vi "Teleop.vi"(10 "Match Info":T1={"Autonomous Elapsed Seconds"=0.0, "TeleOp Elapsed Seconds"=0.0, "Disabled Elapsed Seconds"=0.0, "Visited Autonomous"=FALSE, "Visited TeleOp"=FALSE, "Visited Disabled"=FALSE, "Autonomous Settings"={"Autonomous Style"=enum."Independent", "VI Refnum"=refnum}}, 11 "Call Context":T2) -> ()   [LabVIEW 2016]
doc: "This VI is called for each TeleOp packet received from the DS where the robot is not disabled. It is often used to read from the joysticks and update I/O or to update setpoints for timed control loops. It should complete and return within 20 milliseconds or it may miss DS packets."
uses:
  <vilib>/Rock Robotics/WPI/DriverStation/WPI_DriverStationDerivedRobotMode.ctl
  <vilib>/Rock Robotics/WPI/DriverStation/WPI_DriverStationMatch Info.ctl
  <vilib>/Rock Robotics/WPI/Utilities/WPI_GetSetVariantRefNum.vi
  <vilib>/Rock Robotics/Network Tables/NT Write Boolean Array.vi
  <vilib>/Rock Robotics/Network Tables/NT Write Numeric Array.vi
  <vilib>/Rock Robotics/WPI/RobotDrive/WPI_RobotDriveMecanumDrive_Cartesian.vi
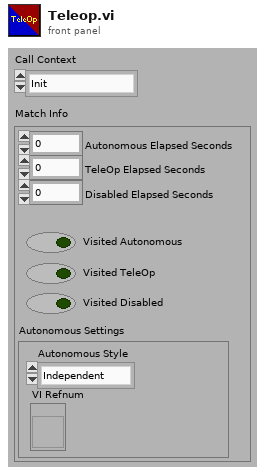
[diagram p1: front panel]
types:
  T1 = typedef "WPI_DriverStationMatch Info.ctl" = cluster{"Autonomous Elapsed Seconds":dbl, "TeleOp Elapsed Seconds":dbl, "Disabled Elapsed Seconds":dbl, "Visited Autonomous":bool, "Visited TeleOp":bool, "Visited Disabled":bool, "Autonomous Settings":cluster{"Autonomous Style":enum16{"Iterative", "Independent"}, "VI Refnum":refnum<vi>}}
  T2 = typedef "WPI_DriverStationDerivedRobotMode.ctl" = enum16{"Init", "Execute", "Stop"}
  T3 = typedef "WPI_JoystickDevRef.ctl" = cluster{"Device":T4}
  T4 = typedef "WPI_JoystickDeviceEnum.ctl" = enum16{"USB 0", "USB 1", "USB 2", "USB 3", "USB 4", "USB 5"}
  T5 = typedef "WPI_RobotDriveDevRef.ctl" = cluster{"DevStatus":errorcluster, "Motors[]":T6[], "Square Inputs":bool, "Max Output":dbl}
  T6 = typedef "WPI_MotorControlDeviceRef.ctl" = cluster{"DeviceStatus":errorcluster, "Type":T7, "PWM":cluster{"PWM Channel":T8, "DeadBand":T9}, "CAN":cluster{"Device Number":u8, "SetOutput VI Ref":variant, "GetOutput VI Ref":variant, "Enable VI Ref":variant, "Disable VI Ref":variant, "Data":variant}, "Invert":bool}
  T7 = typedef "WPI_MotorControlType.ctl" = enum16{"PWM", "CAN"}
  T8 = typedef "FPGA_DIOPWMChannel.ctl" = enum8{"PWM 0", "PWM 1", "PWM 2", "PWM 3", "PWM 4", "PWM 5", "PWM 6", "PWM 7", "PWM 8", "PWM 9", "PWM MXP 0", "PWM MXP 1", "PWM MXP 2", "PWM MXP 3", "PWM MXP 4", "PWM MXP 5", "PWM MXP 6", "PWM MXP 7", "PWM MXP 8", "PWM MXP 9", "Invalid"}
  T9 = typedef "WPI_PWMDeadband.ctl" = cluster{"Name":string, "maxPositivePwm":i32, "minPositivePwm":i32, "centerPwm":i32, "maxNegativePwm":i32, "minNegativePwm":i32, "angularRange":u16}
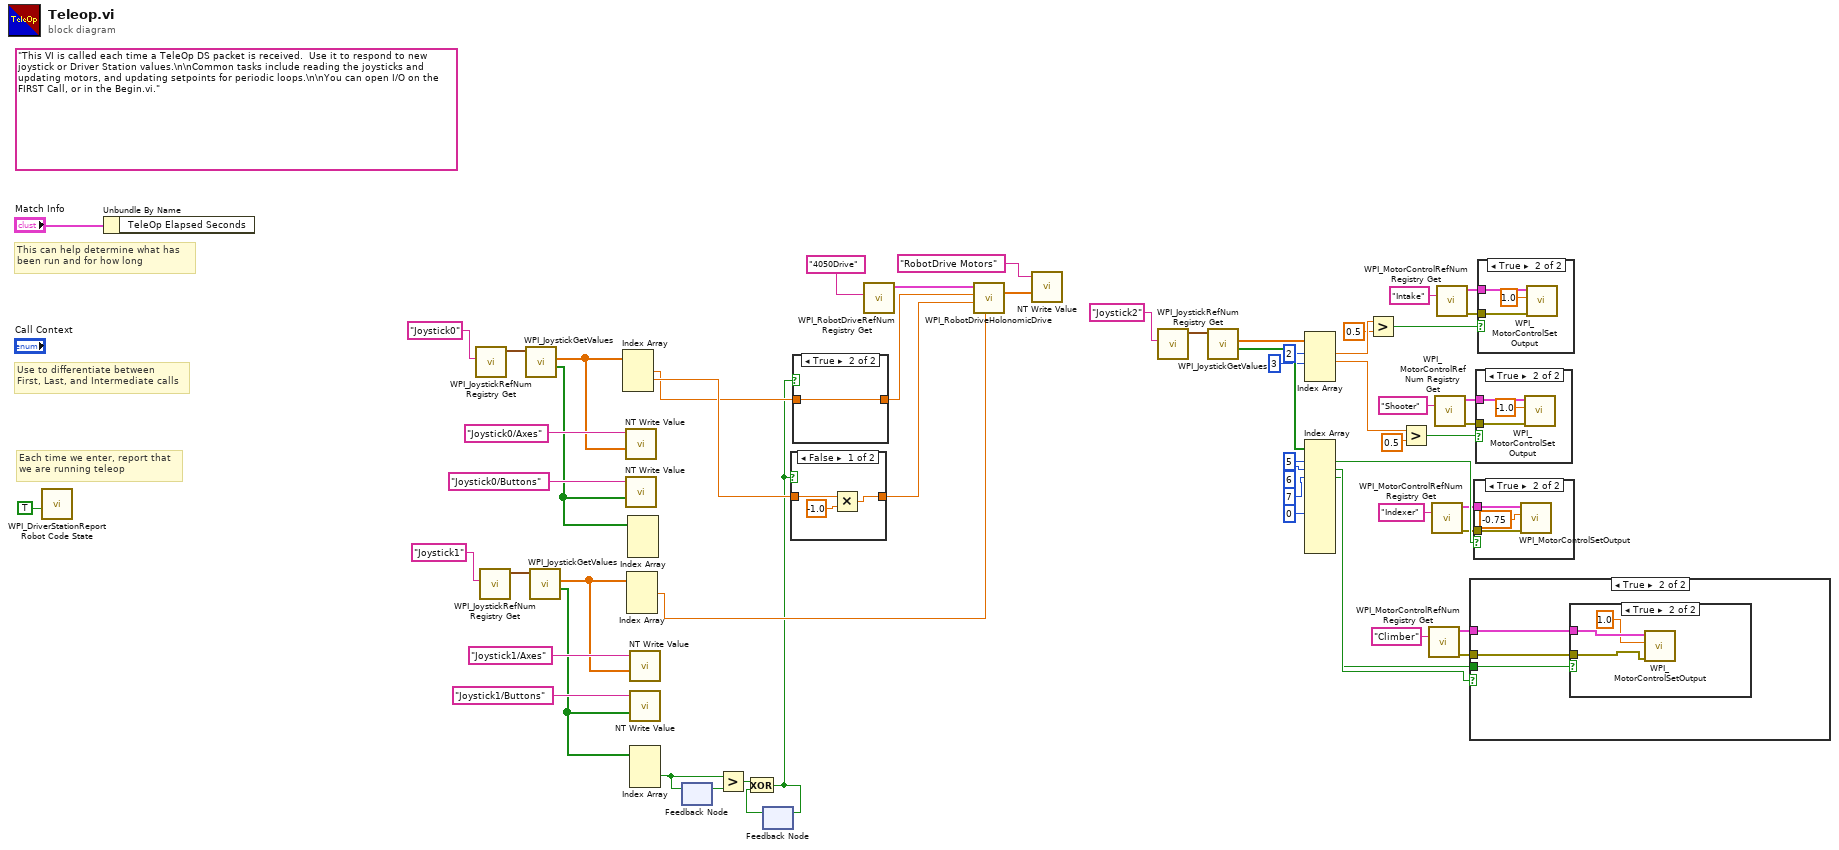
[diagram p0: block diagram]
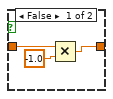
[diagram p2: hidden frame]
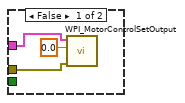
[diagram p4: hidden frame]
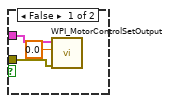
[diagram p5: hidden frame]
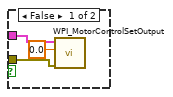
[diagram p6: hidden frame]
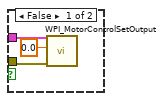
[diagram p7: hidden frame]
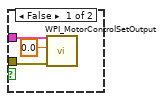
[diagram p8: hidden frame]
diagram:
  (unwired) "This VI is called each time a TeleOp DS packet is received.  Use it to respond to new joystick or Driver Station values.\n\nCommon tasks include reading the joysticks and updating motors, and updating setpoints for periodic loops.\n\nYou can open I/O on the FIRST Call, or in the Begin.vi."
  # "Each time we enter, report that\nwe are running teleop"
  # "Use to differentiate between\nFirst, Last, and Intermediate calls"
  # "This can help determine what has\nbeen run and for how long"
  n1 = call <vilib>:"WPI_DriverStationReport Robot Code State.vi"("TeleOp"=TRUE ("Autonomous")) -> ()  [unwired: 10 in, 1 out]
  n2 = Unbundle By Name("Match Info") -> ()  [unwired: 1 out]
  n3 = call <vilib>:"WPI_JoystickRefNum Registry Get.vi"("refnum name"="Joystick0") -> ("JoystickDevRef"=w55:T3)  [unwired: 1 in, 9 out]
  n4 = call <vilib>:"WPI_JoystickRefNum Registry Get.vi"("refnum name"="Joystick1") -> ("JoystickDevRef"=w47:T3)  [unwired: 1 in, 9 out]
  n5 = call <vilib>:"WPI_JoystickGetValues.vi"("JoystickDevRef"=w55) -> ("Buttons"=w39:bool[], "Axes"=w52:dbl[])  [unwired: 6 in, 3 out]
  n6 = call <vilib>:"WPI_JoystickGetValues.vi"("JoystickDevRef"=w47) -> ("Buttons"=w16:bool[], "Axes"=w45:dbl[])  [unwired: 6 in, 3 out]
  n7 = Index Array(array=w52) -> (element #1=w4:dbl, element #2=w6:dbl)  [unwired: 3 in, 1 out]
  n8 = call-poly <vilib>:"NT Write Value.vi"("Numeric Array"=w52, "Name"="Joystick0/Axes") -> ()  [unwired: 9 in, 1 out]
  n9 = call-poly <vilib>:"NT Write Value.vi"("Boolean Array"=w39, "Name"="Joystick0/Buttons") -> ()  [unwired: 9 in, 1 out]
  n10 = Index Array(array=w45) -> (element #1=w3:dbl)  [unwired: 3 in, 2 out]
  n11 = Index Array(array=w39) -> ()  [unwired: 3 in, 3 out]
  n12 = call-poly <vilib>:"NT Write Value.vi"("Numeric Array"=w45, "Name"="Joystick1/Axes") -> ()  [unwired: 9 in, 1 out]
  n13 = call-poly <vilib>:"NT Write Value.vi"("Boolean Array"=w16, "Name"="Joystick1/Buttons") -> ()  [unwired: 9 in, 1 out]
  n14 = Index Array(array=w16) -> (element #2=w15:bool)  [unwired: 3 in, 2 out]
  n15 = feedback-in #1(w15) -> ()
  n16 = feedback #1() -> (w14:bool)  [unwired: 1 in]
  n17 = Greater?(x=w15, y=w14) -> (0:w13:bool)
  n18 = feedback #2() -> (w12:bool)  [unwired: 1 in]
  n19 = Exclusive Or(1:w12, 2:w13) -> (0:w2:bool)
  n20 = feedback-in #2(w2) -> ()
  n21 = case shown="False" w2 {
    tunnel: [w62 w63] -> w7
    tunnel: w6 -> [w61 w63]
    frame False {
      n22 = Multiply(x=w61, y=-1.0) -> (x*y=w62:dbl)
    }
    frame True {
    }
  }
  n23 = case shown="True" w2 {
    tunnel: [w66 w67] -> w5
    tunnel: w4 -> [w65 w67]
    frame False {
      n24 = Multiply(x=w65, y=-1.0) -> (x*y=w66:dbl)
    }
    frame True {
    }
  }
  n25 = call <vilib>:"WPI_RobotDriveRefNum Registry Get.vi"("refnum name"="4050Drive") -> ("RobotDriveDevRef"=w57:T5)  [unwired: 1 in, 9 out]
  n26 = call-poly <vilib>:"WPI_RobotDriveHolonomicDrive.vi"("Rotation"=w3, "Y"=w7, "X"=w5, "RobotDriveDevRef"=w57) -> ("Motor Values"=w50:dbl[])  [unwired: 5 in, 2 out]
  n27 = call-poly <vilib>:"NT Write Value.vi"("Numeric Array"=w50, "Name"="RobotDrive Motors") -> ()  [unwired: 9 in, 1 out]
  n28 = call <vilib>:"WPI_JoystickRefNum Registry Get.vi"("refnum name"="Joystick2") -> ("JoystickDevRef"=w42:T3)  [unwired: 1 in, 9 out]
  n29 = call <vilib>:"WPI_JoystickGetValues.vi"("JoystickDevRef"=w42) -> ("Buttons"=w40:bool[], "Axes"=w41:dbl[])  [unwired: 6 in, 3 out]
  n30 = Index Array(array=w41, index #1=2 ("index"), index #2=3 ("index")) -> (element #1=w37:dbl, element #2=w25:dbl)  [unwired: 2 in, 2 out]
  n31 = Index Array(array=w40, index #1=5 ("index"), index #2=6 ("index"), index #3=7 ("index"), index #4=0 ("index")) -> (element #1=w23:bool, element #2=w11:bool, element #3=w8:bool)  [unwired: 8 in, 9 out]
  n32 = Greater?(x=w37, y=0.5) -> (0:w35:bool)
  n33 = Greater?(x=w25, y=0.5) -> (0:w26:bool)
  n34 = call <vilib>:"WPI_MotorControlRefNum Registry Get.vi"("refnum name"="Climber") -> ("error out"=w17:errorcluster, "MotorControlDevRef"=w18:T6)  [unwired: 9 in]
  n35 = call <vilib>:"WPI_MotorControlRefNum Registry Get.vi"("refnum name"="Indexer") -> ("error out"=w20:errorcluster, "MotorControlDevRef"=w21:T6)  [unwired: 9 in]
  n36 = call <vilib>:"WPI_MotorControlRefNum Registry Get.vi"("refnum name"="Shooter") -> ("error out"=w28:errorcluster, "MotorControlDevRef"=w29:T6)  [unwired: 9 in]
  n37 = call <vilib>:"WPI_MotorControlRefNum Registry Get.vi"("refnum name"="Intake") -> ("error out"=w32:errorcluster, "MotorControlDevRef"=w33:T6)  [unwired: 9 in]
  n38 = case shown="True" w11 {
    tunnel: w18 -> [w69 w73]
    tunnel: w17 -> [w68 w72]
    tunnel: w8 -> [_ w71]
    frame False {
      n39 = call <vilib>:"WPI_MotorControlSetOutput.vi"("error in (no error)"=w68, "Output"=0.0, "MotorControlDevRef"=w69) -> ()  [unwired: 6 in, 3 out]
    }
    frame True {
      n40 = case shown="True" w71 {
        tunnel: w73 -> [w76 w79]
        tunnel: w72 -> [w75 w78]
        frame False {
          n41 = call <vilib>:"WPI_MotorControlSetOutput.vi"("error in (no error)"=w75, "Output"=0.0, "MotorControlDevRef"=w76) -> ()  [unwired: 6 in, 3 out]
        }
        frame True {
          n42 = call <vilib>:"WPI_MotorControlSetOutput.vi"("error in (no error)"=w78, "Output"=1.0, "MotorControlDevRef"=w79) -> ()  [unwired: 6 in, 3 out]
        }
      }
    }
  }
  n43 = case shown="True" w23 {
    tunnel: w21 -> [w82 w84]
    tunnel: w20 -> [w81 w83]
    frame False {
      n44 = call <vilib>:"WPI_MotorControlSetOutput.vi"("error in (no error)"=w81, "Output"=0.0, "MotorControlDevRef"=w82) -> ()  [unwired: 6 in, 3 out]
    }
    frame True {
      n45 = call <vilib>:"WPI_MotorControlSetOutput.vi"("error in (no error)"=w83, "Output"=-0.75, "MotorControlDevRef"=w84) -> ()  [unwired: 6 in, 3 out]
    }
  }
  n46 = case shown="True" w26 {
    tunnel: w29 -> [w88 w91]
    tunnel: w28 -> [w87 w90]
    frame False {
      n47 = call <vilib>:"WPI_MotorControlSetOutput.vi"("error in (no error)"=w87, "Output"=0.0, "MotorControlDevRef"=w88) -> ()  [unwired: 6 in, 3 out]
    }
    frame True {
      n48 = call <vilib>:"WPI_MotorControlSetOutput.vi"("error in (no error)"=w90, "Output"=-1.0, "MotorControlDevRef"=w91) -> ()  [unwired: 6 in, 3 out]
    }
  }
  n49 = case shown="True" w35 {
    tunnel: w33 -> [w94 w97]
    tunnel: w32 -> [w93 w96]
    frame False {
      n50 = call <vilib>:"WPI_MotorControlSetOutput.vi"("error in (no error)"=w93, "Output"=0.0, "MotorControlDevRef"=w94) -> ()  [unwired: 6 in, 3 out]
    }
    frame True {
      n51 = call <vilib>:"WPI_MotorControlSetOutput.vi"("error in (no error)"=w96, "Output"=1.0, "MotorControlDevRef"=w97) -> ()  [unwired: 6 in, 3 out]
    }
  }
